vi "initialize.vi"(0 "HGF_DSCVarManager":refnum<class "HGF_DSCVarManager.lvclass">, 3 "initializationData":variant, 5 "error in (no error)":errorcluster, 7 "binaryString":string, 8 "I8 Array":i8[](array[numeric]), 9 "prependSize? (T)":bool, 11 "byteOrder (0:big-endian, network order)":T1(ring)) -> (14 "dup HGF_DSCVarManager":refnum<class "HGF_DSCVarManager.lvclass">, 17 "found?":bool, 19 "error out":errorcluster)   [LabVIEW 2012, in "HGF_DSC.lvlib" / "HGF_DSCVarManager.lvclass"]
doc: "This is a dynamic dispatch VI to be implemented by child classes to initialize their attributes.\n\n<B>Recommendation:</B> Use Variant for initialization data."
uses:
  HGF_DSCVarManager.lvclass
  HGF_BaseClasses/HGF_Visitable/HGF_Visitable.lvclass
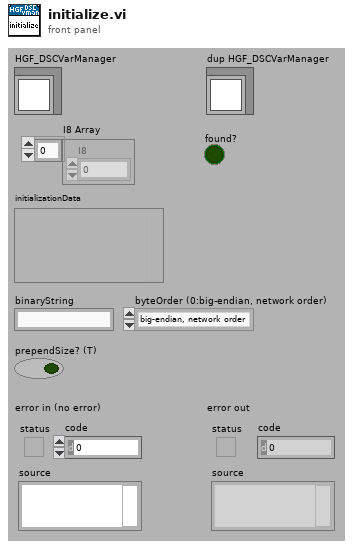
[diagram p1: front panel]
types:
  T1 = enum16{"big-endian, network order", "native, host order", "little-endian"}
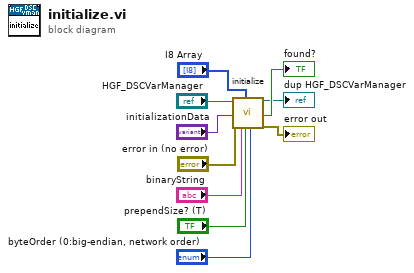
[diagram p0: block diagram]
diagram:
  n1 = call-parent "initialize.vi"("HGF_Base"="HGF_DSCVarManager", "initializationData"="initializationData", "error in (no error)"="error in (no error)", "binaryString"="binaryString", "I8 Array"="I8 Array", "prependSize? (T)"="prependSize? (T)", "byteOrder (0:big-endian, network order)"="byteOrder (0:big-endian, network order)") -> ("dup HGF_Base"=→"dup HGF_DSCVarManager":refnum<class "HGF_DSCVarManager.lvclass">, "found?"=→"found?":bool, "error out"=→"error out":errorcluster)  [unwired: 10 out]
